vi "主画面.vi"() -> ()   [LabVIEW 2016]
uses:
  <vilib>/Utility/miscctls.llb/LVPointTypeDef.ctl
  <vilib>/Utility/miscctls.llb/LVRectTypeDef.ctl
  data/FreeMem.dll
  API/update/update.lvlib
panel:
  out "title":string="浮标多参数水质监测仪"
  out "SN":string="系列号"
  in  "关于":bool
  in  "全屏":T1
  out "站点名称":string="站点名称"
  out "时间显示":string="2017-05-09 10:50:42"
  in  "主画面菜单":enum32{"首页", "数据查询", "运维调试", "环境动力", "系统设置"}(xcontrol)
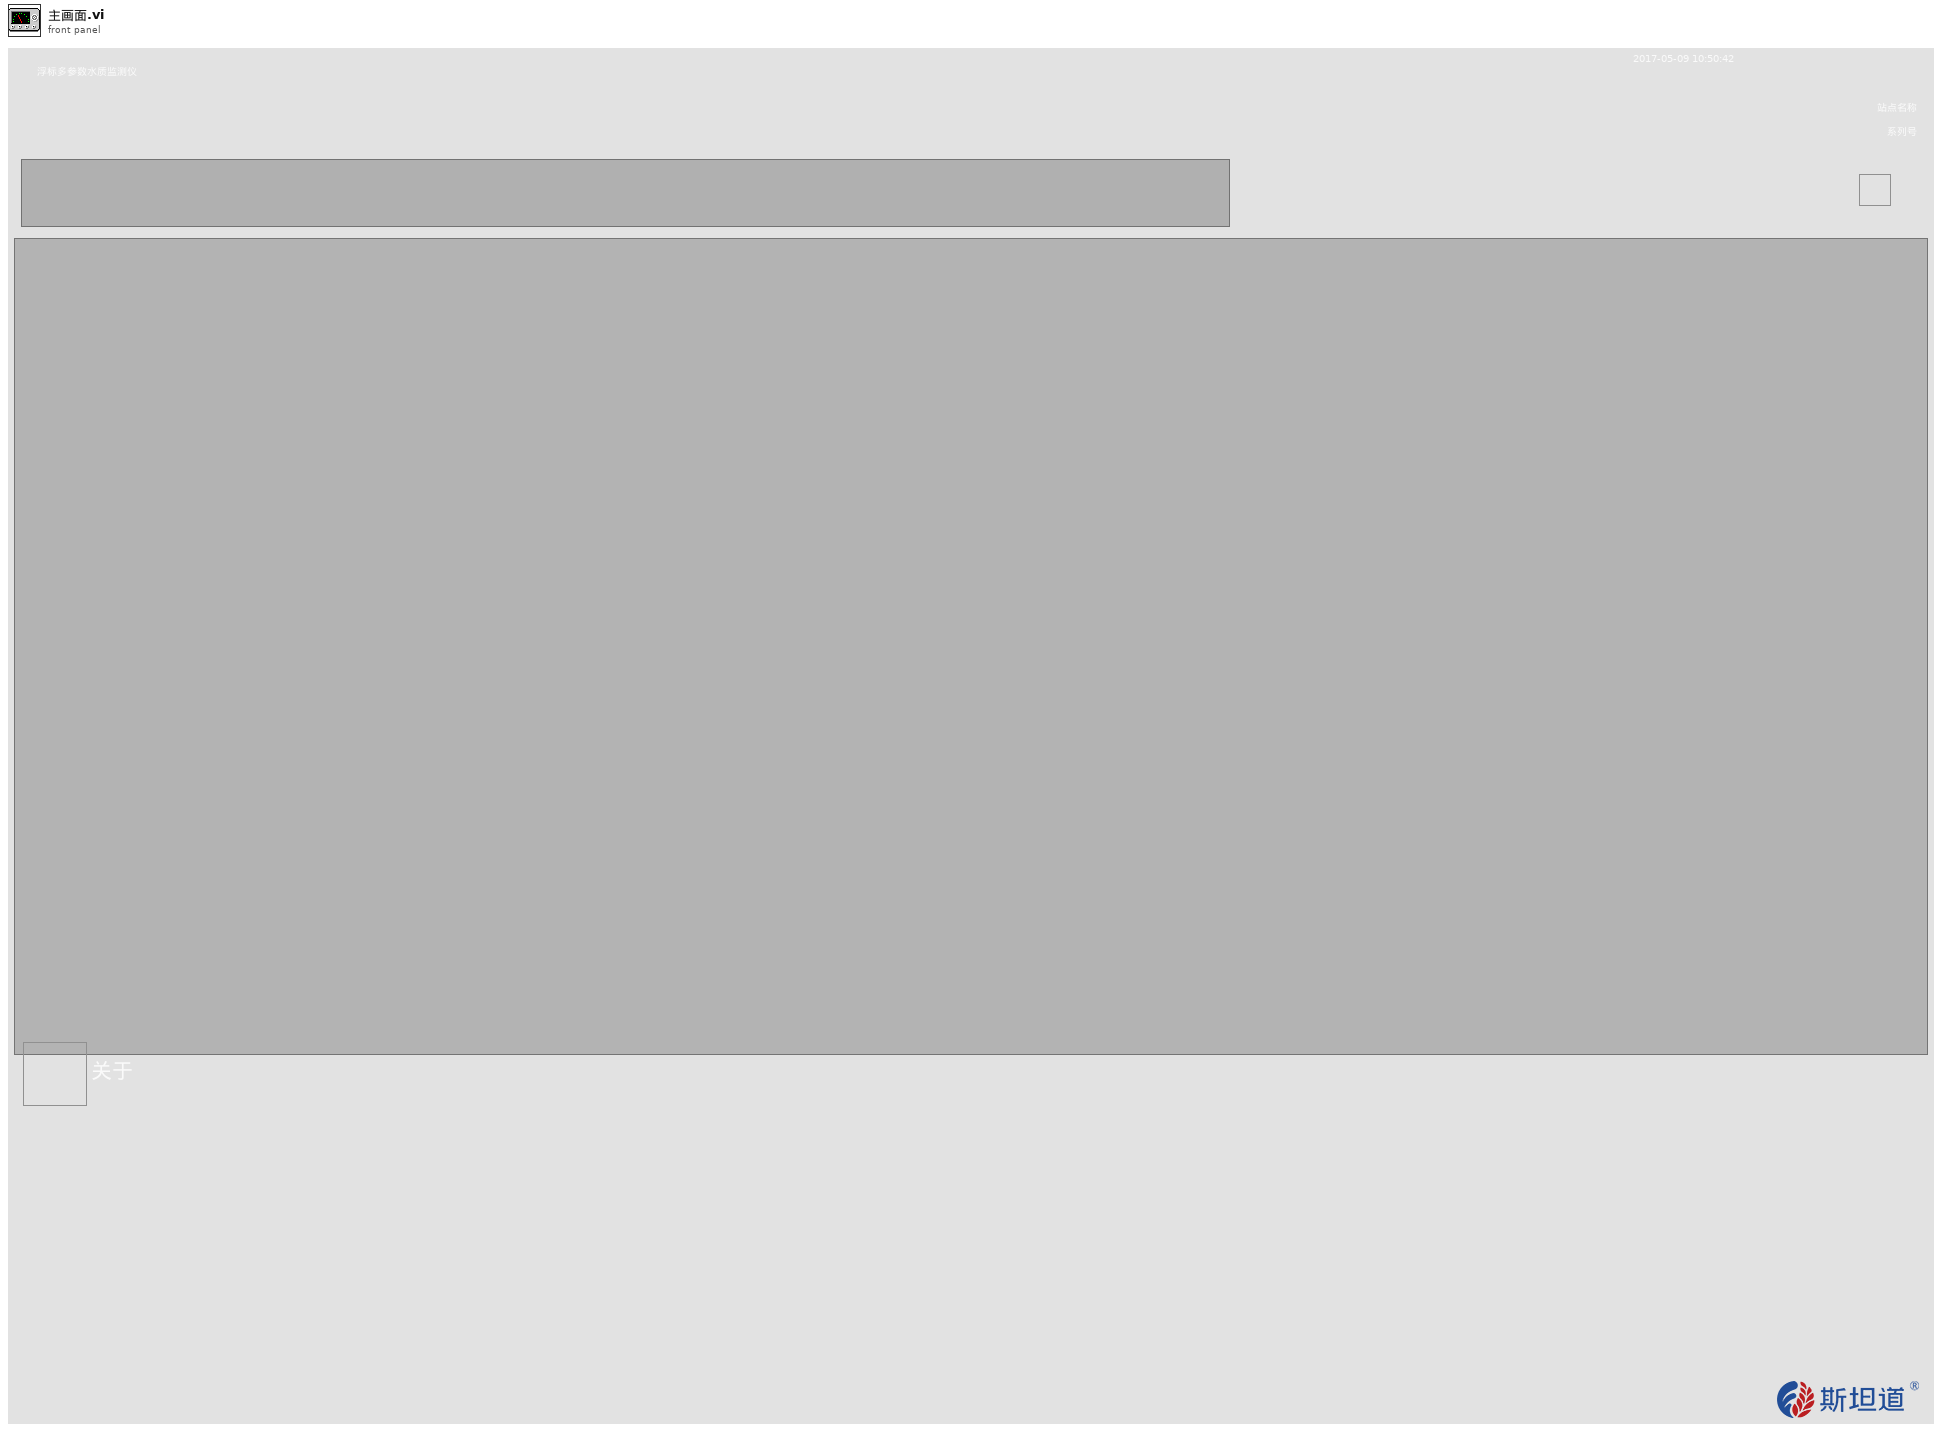
[diagram p1: front panel]
types:
  T1 = typedef "全屏按钮.ctl" = bool
  T2 = typedef "LVPointTypeDef.ctl" = cluster{"Horizontal":i16, "Vertical":i16}
  T3 = cluster{"时间标识":timestamp, "设备":string, "日志信息":string, "流程参数":string}
  T4 = enum32{"Bad", "Idle", "Run top level", "Running"}
  T5 = typedef "LVRectTypeDef.ctl" = cluster{"Left":i16, "Top":i16, "Right":i16, "Bottom":i16}
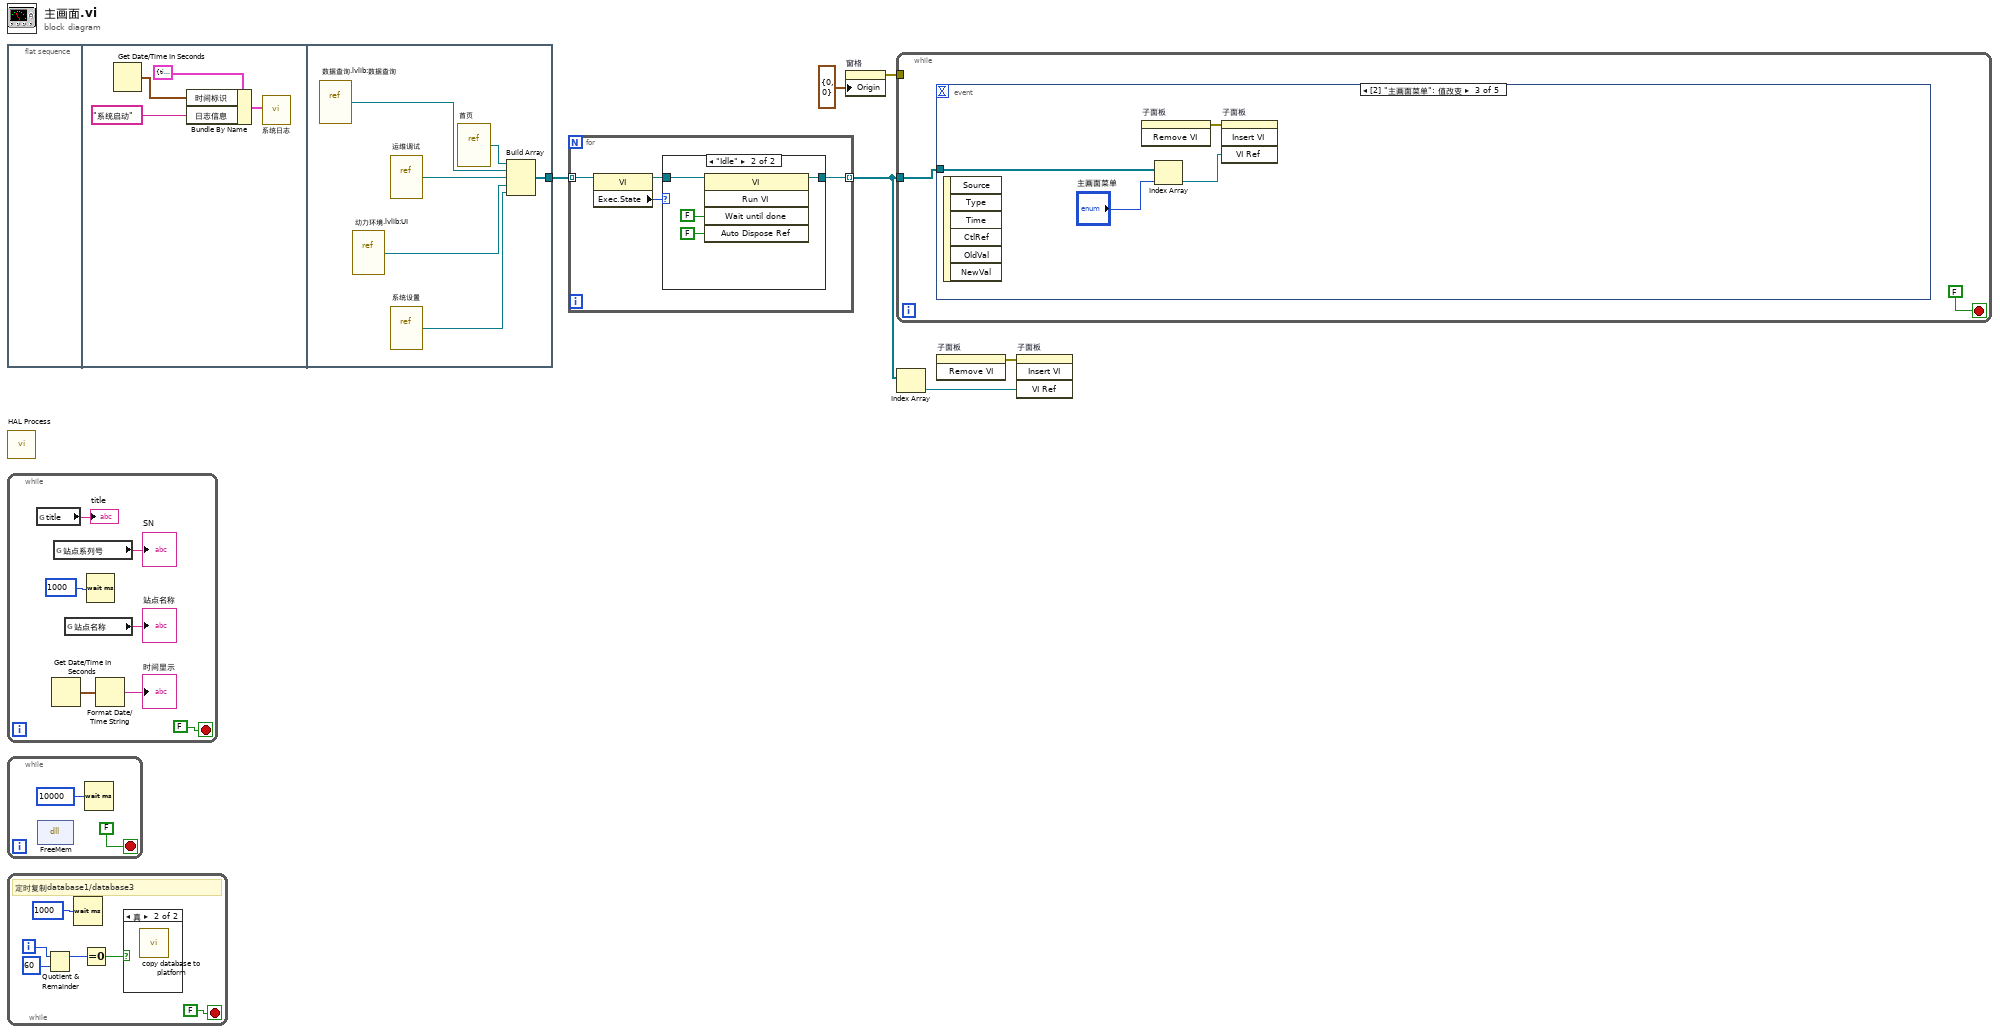
[diagram p0: block diagram]
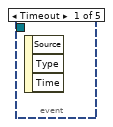
[diagram p4: hidden frame]
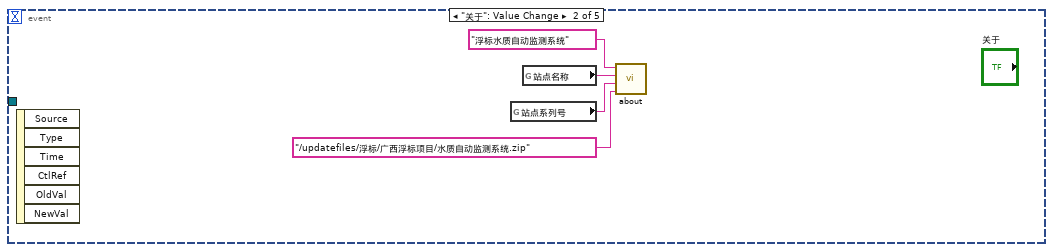
[diagram p5: hidden frame]
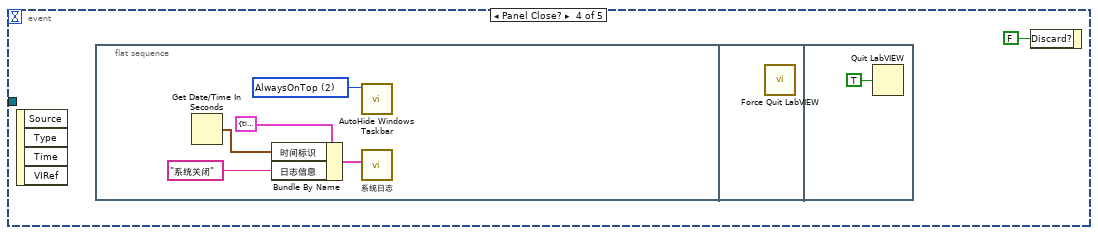
[diagram p6: hidden frame]
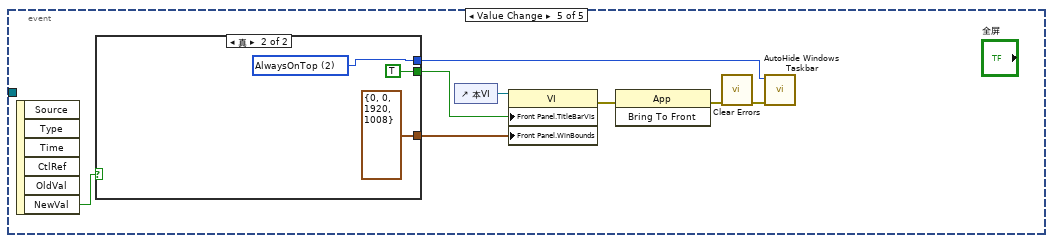
[diagram p7: hidden frame]
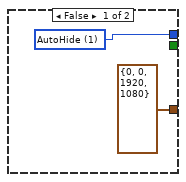
[diagram p8: hidden frame]
diagram:
  n1 = flat-sequence {
    tunnel: [w12] -> w3
    frame #0 {
    }
    frame #1 {
      n2 = Get Date/Time In Seconds() -> (seconds since 1Jan1904=w8:timestamp)
      n3 = Bundle By Name(cluster=T3 {"时间标识"=timestamp(0 s since 1904-01-01), "设备"="系统", "日志信息"="", "流程参数"=""} ("data in"), "时间标识"=w8, "日志信息"="系统启动") -> (w9:T3)
      n4 = call "系统日志.vi"("data in"=w9) -> ()  [unwired: 11 in]
    }
    frame #2 {
      n5 = vi-ref "数据查询.lvlib:数据查询.vi"() -> (w14:refnum<vi>)
      n6 = vi-ref "动力环境.lvlib:UI.vi"() -> (w11:refnum<vi>)
      n7 = vi-ref "运维调试.vi"() -> (w15:refnum<vi>)
      n8 = vi-ref "系统设置.vi"() -> (w16:refnum<vi>)
      n9 = vi-ref "首页.vi"() -> (w13:refnum<vi>)
      n10 = Build Array(w13, w14, w15, w11, w16) -> (w12:refnum<vi>[])
    }
  }
  n11 = call "HAL Process.vi"() -> ()  [unwired: 12 in]
  n12 = while {
    stop <- FALSE stop-if-true
    n13 = global read "系统设置全局变量.vi" "title"() -> (→"title":string)
    n14 = Get Date/Time In Seconds() -> (seconds since 1Jan1904=w20:timestamp)
    n15 = global read "系统设置全局变量.vi" "站点系列号"() -> (→"SN":string)
    n16 = global read "系统设置全局变量.vi" "站点名称"() -> (→"站点名称":string)
    n17 = Wait (ms)(milliseconds to wait=u32 1000 ("等待时间（毫秒）")) -> ()  [unwired: 1 out]
    n18 = Format Date/Time String(seconds (now)=w20) -> (date/time string=→"时间显示":string)  [unwired: 2 in]
  }
  n19 = while {
    stop <- FALSE stop-if-true
    n20 = dll-call lib="PTH2:abs F广西浮标项目\nSourceCodedataFreeMem.dll" fn="FreeMem"() -> ()  [unwired: 4 in, 2 out]
    n21 = Wait (ms)(milliseconds to wait=u32 10000 ("等待时间（毫秒）")) -> ()  [unwired: 1 out]
  }
  n22 = while {
    i -> [w29]
    stop <- FALSE stop-if-true
    # "定时复制database1/database3"
    n23 = Quotient & Remainder(x=w29, y=60) -> (x-y*floor(x/y)=w27:i32)  [unwired: 1 out]
    n24 = Wait (ms)(milliseconds to wait=u32 1000 ("等待时间（毫秒）")) -> ()  [unwired: 1 out]
    n25 = Equal To 0?(x=w27) -> (x = 0?=w26:bool)
    n26 = case shown="真" w26 {
      frame False {
      }
      frame True {
        n27 = call "copy database to platform.vi"() -> ()  [unwired: 12 in]
      }
    }
  }
  n28 = for {
    tunnel: w3 -> [w35] mode=indexing
    tunnel: [w32] -> w5 mode=indexing
    n29 = property class="VI"(reference=w35) -> (reference out=w33:refnum<vi>, "Exec.State"=w34:T4)  [unwired: 1 in, 1 out]
    n30 = case shown="\"Idle\"" w34 {
      tunnel: w33 -> [w36 w38]
      tunnel: [w36 w37] -> w32
      frame "Bad", Default {
      }
      frame "Idle" {
        n31 = invoke class="VI" method="Run VI"(reference=w38, "Wait until done"=FALSE ("结束前等待"), "Auto Dispose Ref"=FALSE ("自动销毁引用")) -> (reference out=w37:refnum<vi>)  [unwired: 2 in, 4 out]
      }
    }
  }
  n32 = property on="窗格" class="Pane"("Origin"=T2 {"Horizontal"=0, "Vertical"=0} ("原点")) -> (error out=w1:errorcluster)  [unwired: 2 in, 1 out]
  n33 = while {
    tunnel: w5 -> [w41]
    tunnel: w1 -> [_]
    stop <- FALSE stop-if-true
    n34 = event shown="[2] \"主画面菜单\": 值改变" {
      selector: _ -> [_ _ _ _ _]
      dyn-events: _ -> [_ _ _ _ _]
      timeout: _ -> [_ _ _ _ _]
      tunnel: w41 -> [_ _ w49 _ _]
      event Timeout {
        n35 = event-data() -> ()  [unwired: 1 in, 3 out]
      }
      event "关于": Value Change {
        n36 = event-data() -> ()  [unwired: 1 in, 6 out]
        n37 = global read "系统设置全局变量.vi" "站点系列号"() -> (w45:string)
        n38 = global read "系统设置全局变量.vi" "站点名称"() -> (w44:string)
        n39 = call "about.vi"("更新包远端地址"="/updatefiles/浮标/广西浮标项目/水质自动监测系统.zip", "SN输入"=w45, "站点名称输入"=w44, "应用程序名称输入"="浮标水质自动监测系统") -> ()  [unwired: 8 in]
      }
      event "主画面菜单": Value Change {
        n40 = event-data() -> ()  [unwired: 1 in, 6 out]
        n41 = invoke on="子面板" class="SubPnl" method="Remove VI"() -> (error out=w47:errorcluster)  [unwired: 3 in, 2 out]
        n42 = Index Array(array=w49, index="主画面菜单") -> (element=w48:refnum<vi>)
        n43 = invoke on="子面板" class="SubPnl" method="Insert VI"(error in=w47, "VI Ref"=w48) -> ()  [unwired: 2 in, 4 out]
      }
      event Panel Close? {
        n44 = event-data() -> ()  [unwired: 1 in, 4 out]
        n45 = flat-sequence {
          frame #0 {
            w52 = u8 2 items=["AutoHide"=1, "AlwaysOnTop"=2] ("Operation")
            n46 = Get Date/Time In Seconds() -> (seconds since 1Jan1904=w55:timestamp)
            n47 = Bundle By Name(cluster=T3 {"时间标识"=timestamp(0 s since 1904-01-01), "设备"="系统", "日志信息"="", "流程参数"=""} ("data in"), "时间标识"=w55, "日志信息"="系统关闭") -> (w54:T3)
            n48 = call "AutoHide Windows Taskbar.vi"("Operation"=w52) -> ()  [unwired: 6 in, 1 out]
            n49 = call "系统日志.vi"("data in"=w54) -> ()  [unwired: 11 in]
          }
          frame #1 {
            n50 = call "Force Quit LabVIEW.vi"() -> ()  [unwired: 10 in, 2 out]
          }
          frame #2 {
            n51 = Quit LabVIEW(quit? (T)=TRUE ("退出？(T)")) -> ()
          }
        }
        n52 = event-data("Discard?"=FALSE ("放弃？")) -> ()  [unwired: 1 in, 1 out]
      }
      event Value Change {
        n53 = event-data() -> ("NewVal"=w65:T1)  [unwired: 1 in, 5 out]
        n54 = case shown="真" w65 {
          tunnel: [w67 w70] -> w64
          tunnel: [T5 {"Left"=0, "Top"=0, "Right"=1920, "Bottom"=1080} ("前面板窗口:窗口边界") T5 {"Left"=0, "Top"=0, "Right"=1920, "Bottom"=1008} ("前面板窗口:窗口边界")] -> w61
          tunnel: [_ TRUE] -> w59
          frame False {
            w67 = u8 1 items=["AutoHide"=1, "AlwaysOnTop"=2] ("Operation")
          }
          frame True {
            w70 = u8 2 items=["AutoHide"=1, "AlwaysOnTop"=2] ("Operation")
          }
        }
        n55 = control-ref of="本VI"() -> (w63:refnum<vi>)
        n56 = property class="VI"(reference=w63, "Front Panel.TitleBarVis"=w59, "Front Panel.WinBounds"=w61) -> (error out=w62:errorcluster)  [unwired: 1 in, 1 out]
        n57 = invoke class="App" method="Bring To Front"(error in=w62) -> (error out=w60:errorcluster)  [unwired: 2 in, 2 out]
        n58 = call <vilib>:"Clear Errors.vi"("error in (no error)"=w60) -> ("error out"=w58:errorcluster)  [unwired: 5 in, 1 out]
        n59 = call "AutoHide Windows Taskbar.vi"("error in (no error)"=w58, "Operation"=w64) -> ()  [unwired: 5 in, 1 out]
      }
    }
  }
  n60 = Index Array(array=w5) -> (element=w4:refnum<vi>)  [unwired: 1 in]
  n61 = invoke on="子面板" class="SubPnl" method="Remove VI"() -> (error out=w6:errorcluster)  [unwired: 3 in, 2 out]
  n62 = invoke on="子面板" class="SubPnl" method="Insert VI"(error in=w6, "VI Ref"=w4) -> ()  [unwired: 2 in, 4 out]
